vi "Insight_Streaming_Initiate.vi"(8 "error in (no error)":errorcluster) -> (0 "error out":errorcluster, 2 "Data Queue":refnum<queue>, 3 "Streaming VI":refnum<vi>)   [LabVIEW 2015]
panel:
  out "abort error (ignored)":errorcluster
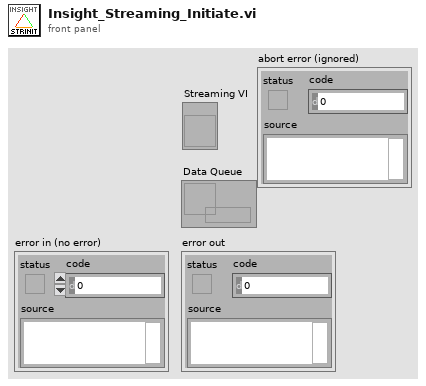
[diagram p1: front panel]
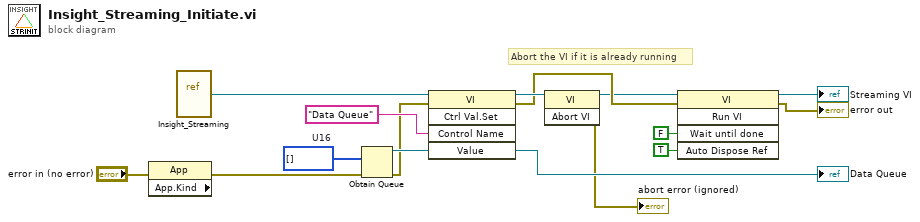
[diagram p0: block diagram]
diagram:
  w9 = u16[] []  # U16
  # "Abort the VI if it is already running"
  n1 = property class="App" props=["App.Kind"](error in="error in (no error)") -> (error out=w6:errorcluster)  [unwired: 1 in, 2 out]
  n2 = vi-ref "Insight_Streaming.vi"() -> (w5:refnum<vi>)
  n3 = Obtain Queue(element data type=w9, error in (no error)=w6) -> (queue out=w12:refnum<queue>, error out=w8:errorcluster)  [unwired: 3 in, 1 out]
  "Data Queue" <- w12
  n4 = invoke class="VI" method="Ctrl Val.Set"(reference=w5, error in=w8, "Control Name"="Data Queue", "Value"=w12) -> (reference out=w4:refnum<vi>, error out=w3:errorcluster)  [unwired: 1 in, 3 out]
  n5 = invoke class="VI" method="Abort VI"(reference=w4) -> (reference out=w1:refnum<vi>, error out=→"abort error (ignored)":errorcluster)  [unwired: 2 in, 1 out]
  n6 = invoke class="VI" method="Run VI"(reference=w1, error in=w3, "Wait until done"=FALSE ("Wait Until Done"), "Auto Dispose Ref"=TRUE ("Auto Dispose Reference")) -> (reference out=→"Streaming VI":refnum<vi>, error out=→"error out":errorcluster)  [unwired: 1 in, 3 out]
